vi "Hash.vi"(8 "error in (no error)":errorcluster, 10 "Message":string, 11 "SHA-256 in":refnum<class "SHA-256.lvclass">) -> (0 "error out":errorcluster, 2 "Hash":string, 3 "SHA-256 out":refnum<class "SHA-256.lvclass">)   [LabVIEW 2020, in "Crypto.lvlib" / "SHA-256.lvclass"]
uses:
  SHA-256.lvclass
  Compression Iter.vi
  Temp1.vi
  Temp2.vi
  Sigma1.vi
  Choice.vi
  K.vi
  Sigma0.vi
  Major.vi
  Fill W.vi
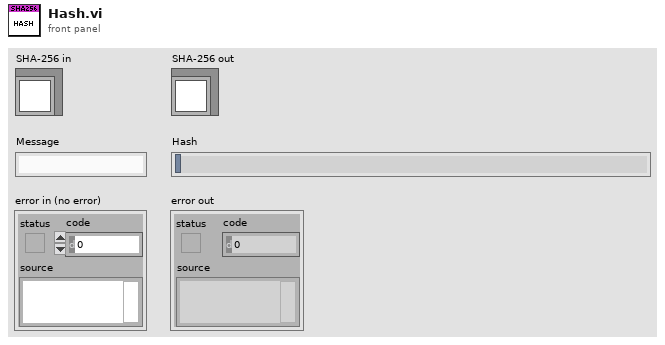
[diagram p1: front panel]
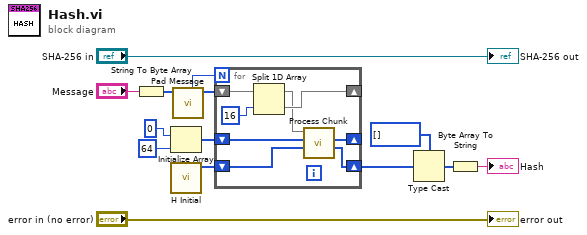
[diagram p0: block diagram]
diagram:
  n1 = String To Byte Array(string="Message") -> (unsigned byte array=w10:u8[])
  n2 = Initialize Array(u32 0 ("element"), 64 ("dimension size")) -> (w7:u32[])
  n3 = call "H Initial.vi"() -> ("H"=w6:u32[])  [unwired: 11 in]
  n4 = call "Pad Message.vi"("Message Byte Array"=w10) -> ("Padded Message"=w9:u32[], "Chunks"=w8:i32)  [unwired: 9 in]
  n5 = for {
    N: w8 -> [_]
    shift-right: [w20] -> _
    shift-left: w9 -> [w22]
    shift-right: [w18] -> _
    shift-left: w7 -> [w19]
    shift-right: [w15] -> w4
    shift-left: w6 -> [w16]
    n6 = Split 1D Array(array=w22, index=16) -> (first subarray=w17:u32[], second subarray=w20:u32[])
    n7 = call "Process Chunk.vi"("H In"=w16, "W In"=w19, "Chunk"=w17) -> ("H"=w15:u32[], "W"=w18:u32[])  [unwired: 7 in]
  }
  n8 = Type Cast(type=u8[] [], x=w4) -> (*(type *) &x=w2:u8[])
  n9 = Byte Array To String(unsigned byte array=w2) -> (string=→"Hash":string)
  "error out" <- "error in (no error)"
  "SHA-256 out" <- "SHA-256 in"
